vi "Umgebung.SolareGewinne.vi"(8 "Error in":errorcluster, 11 "Umgebung in":refnum<data-value>) -> (0 "Error out":errorcluster, 3 "Umgebung out":refnum<data-value>)   [LabVIEW 2016, in "Umgebung.lvclass"]
uses:
  Umgebung.lvclass
  Umgebung.lvclass/Umgebung.ctl
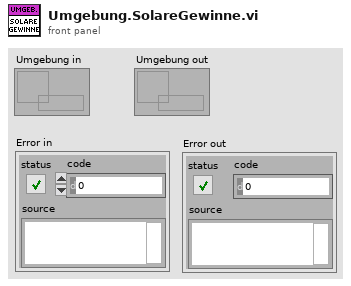
[diagram p1: front panel]
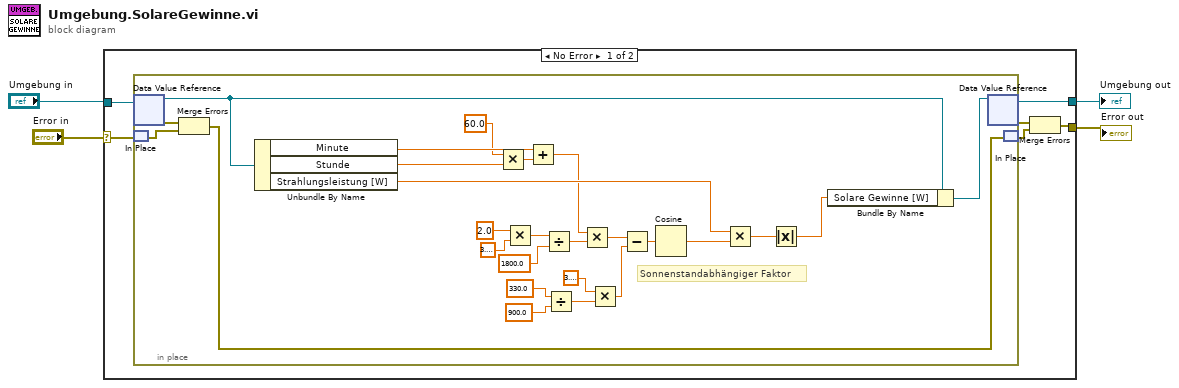
[diagram p0: block diagram]
diagram:
  n1 = case shown="No Error" "Error in" {
    selector: "Error in" -> [w6 w37]
    tunnel: [w7 w37] -> w2
    tunnel: [w10 w38] -> w3
    tunnel: "Umgebung in" -> [w9 w38]
    frame No Error {
      n2 = in-place {
        # "Sonnenstandabhängiger Faktor"
        n3 = in-place-dvr #1(w9) -> (w33:refnum<class "Umgebung.lvclass">, w35:errorcluster)
        n4 = in-place-match #2(w6) -> (w34:errorcluster)
        n5 = Merge Errors(w35, w34) -> (w36:errorcluster)
        n6 = Unbundle By Name(w33) -> ("Minute"=w29:dbl, "Stunde"=w30:dbl, "Strahlungsleistung [W]"=w31:dbl)
        n7 = Multiply(x=60.0, y=w30) -> (x*y=w13:dbl)
        n8 = Multiply(x=2.0, y=3.141592653589793) -> (x*y=w26:dbl)
        n9 = Add(x=w29, y=w13) -> (x+y=w12:dbl)
        n10 = Divide(x=w26, y=1800.0) -> (x/y=w24:dbl)
        n11 = Divide(x=330.0 ("y"), y=900.0) -> (x/y=w22:dbl)
        n12 = Multiply(x=w12, y=w24) -> (x*y=w18:dbl)
        n13 = Multiply(x=3.141592653589793, y=w22) -> (x*y=w17:dbl)
        n14 = Subtract(x=w18, y=w17) -> (x-y=w16:dbl)
        n15 = Cosine(x=w16) -> (cos(x)=w15:dbl)
        n16 = Multiply(x=w31, y=w15) -> (x*y=w11:dbl)
        n17 = Absolute Value(x=w11) -> (abs(x)=w28:dbl)
        n18 = Bundle By Name(cluster=w33, "Solare Gewinne [W]"=w28) -> (w32:refnum<class "Umgebung.lvclass">)
        n19 = in-place-dvr #1(w32) -> (w10:refnum<data-value>, w8:errorcluster)
        n20 = in-place-match #2(w36) -> (w5:errorcluster)
      }
      n21 = Merge Errors(w8, w5) -> (w7:errorcluster)
    }
    frame Error {
    }
  }
  "Umgebung out" <- w3
  "Error out" <- w2
